vi "Installed Distributions [Hemanth].vi"() -> ()   [LabVIEW 2011]
uses:
  <vilib>/registry/registry.llb/Registry SAM.ctl
  <vilib>/registry/registry.llb/Read Registry Value Simple STR.vi
panel:
  in  "Searching in Registry Key and C:\\VM_SETUP\\scriptOut.log":string="SOFTWARE\\National Instruments\\Common\\Installer\\Distributions"
  out "Paths To Installers":string
  out "Dist Names":string[](array[string])
  out "Dist Paths":string[](array[string])
  out "error out":errorcluster
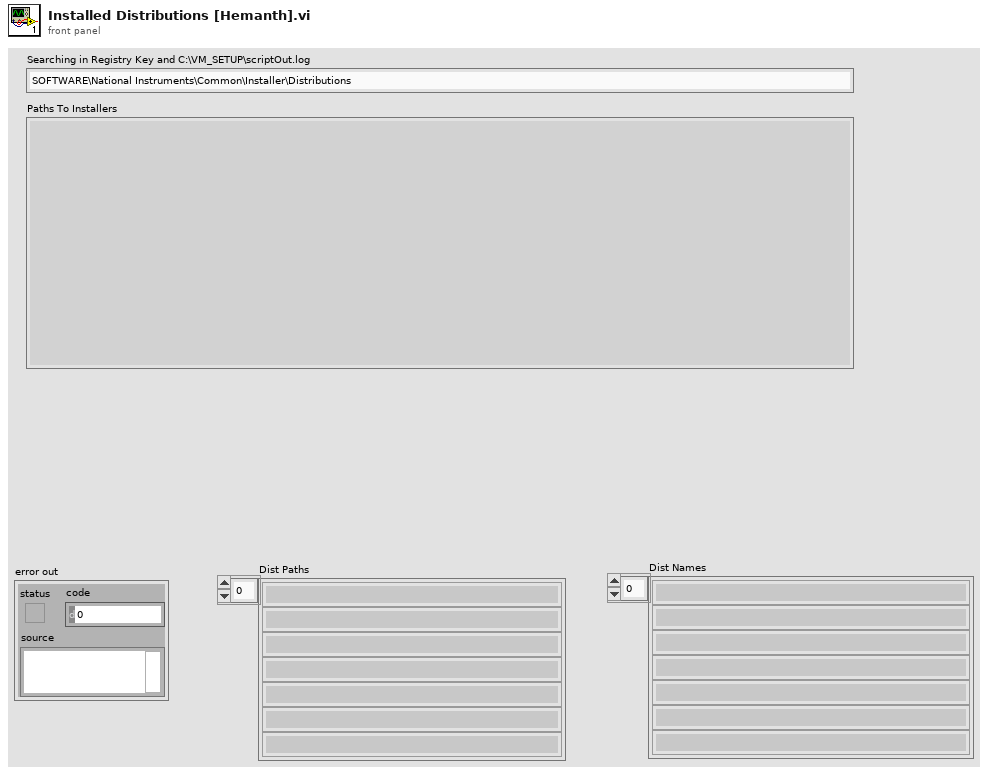
[diagram p1: front panel]
types:
  T1 = typedef "Registry SAM.ctl" = enum32{"KEY_QUERY_VALUE", "KEY_SET_VALUE", "KEY_CREATE_SUB_KEY", "KEY_ENUMERATE_SUB_KEYS", "KEY_NOTIFY", "KEY_CREATE_LINK", "KEY_READ", "KEY_WRITE", "KEY_ALL_ACCESS", "KEY_READ | KEY_WRITE"}
  T2 = typedef "Registry refnum.ctl" = refnum<k1>
  T3 = cluster{"numSubKeys":i32, "maxSubKeyLen":i32, "maxSubKeyClassLen":i32}
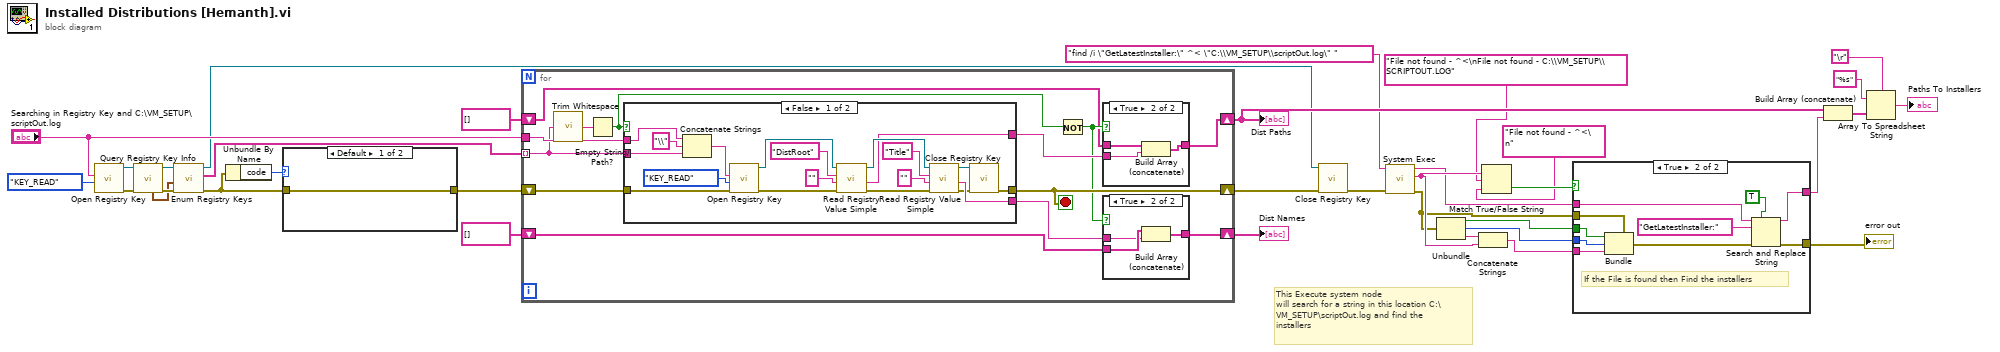
[diagram p0: block diagram]
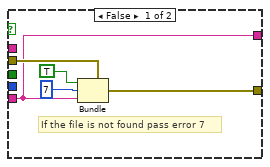
[diagram p2: hidden frame]
diagram:
  # "This Execute system node \nwill search for a string in this location C:\\VM_SETUP\\scriptOut.log and find the installers"
  n1 = call <vilib>:"Open Registry Key.vi"("security access mask (KEY_READ | KEY_WRITE)"=Registry_SAM."KEY_READ", "subkey"="Searching in Registry Key and C:\\VM_SETUP\\scriptOut.log") -> ("error out"=w27:errorcluster, "refnum out"=w29:T2)  [unwired: 8 in]
  n2 = call <vilib>:"Query Registry Key Info.vi"("error in (no error)"=w27, "refnum"=w29) -> ("error out"=w26:errorcluster, "refnum out"=w28:T2, "subkey info"=w25:T3)  [unwired: 5 in, 2 out]
  n3 = call <vilib>:"Enum Registry Keys.vi"("error in (no error)"=w26, "subkey info"=w25, "refnum"=w28) -> ("error out"=w30:errorcluster, "subkeys"=w34:string[], "refnum out"=w15:T2)  [unwired: 6 in]
  n4 = Unbundle By Name(w30) -> ("code"=w31:i32)
  n5 = case shown="Default" w31 {
    tunnel: [w36 _] -> w16
    tunnel: w30 -> [w36 _]
    frame Default {
    }
    frame -605 {
      # "This case is when you have \nless than 100 distirbutions\ninstalled"
    }
  }
  n6 = for {
    tunnel: w34 -> [w44] mode=indexing
    tunnel: "Searching in Registry Key and C:\\VM_SETUP\\scriptOut.log" -> [w49]
    shift-right: [w45] -> w14
    shift-left: w16 -> [w48]
    shift-right: [w39] -> w19
    shift-left: string[] [] ("Array") -> [w40]
    shift-right: [w37] -> w32
    shift-left: string[] [] ("Array") -> [w38]
    stop <- w45 stop-if-true
    n7 = call <vilib>:"Trim Whitespace.vi"("string"=w44) -> ("trimmed string"=w43:string)  [unwired: 1 in]
    n8 = Empty String/Path?(string/path=w43) -> (empty?=w42:bool)
    n9 = case shown="False" w42 {
      tunnel: w49 -> [w75 _]
      tunnel: w44 -> [w74 _]
      tunnel: w48 -> [w71 _]
      tunnel: [w63 _] -> w47
      tunnel: [w59 _] -> w45
      tunnel: [w61 _] -> w46
      frame False {
        n10 = Concatenate Strings(w75, "\\" ("string"), w74) -> (w73:string)
        n11 = call <vilib>:"Open Registry Key.vi"("error in (no error)"=w71, "security access mask (KEY_READ | KEY_WRITE)"=Registry_SAM."KEY_READ", "subkey"=w73) -> ("error out"=w70:errorcluster, "refnum out"=w67:T2)  [unwired: 7 in]
        n12 = call-poly <vilib>:"Read Registry Value Simple.vi"("error in (no error)"=w70, "default data"="", "value"="DistRoot", "refnum"=w67) -> ("error out"=w62:errorcluster, "String/Binary data"=w63:string, "refnum out"=w66:T2)  [unwired: 2 in, 1 out]
        n13 = call-poly <vilib>:"Read Registry Value Simple.vi"("error in (no error)"=w62, "default data"="", "value"="Title", "refnum"=w66) -> ("error out"=w60:errorcluster, "String/Binary data"=w61:string, "refnum out"=w58:T2)  [unwired: 2 in, 1 out]
        n14 = call <vilib>:"Close Registry Key.vi"("error in (no error)"=w60, "refnum"=w58) -> ("error out"=w59:errorcluster)  [unwired: 5 in]
      }
      frame True {
      }
    }
    n15 = Not(x=w42) -> (.not. x?=w41:bool)
    n16 = case shown="True" w41 {
      tunnel: w40 -> [w54 w56]
      tunnel: w47 -> [_ w55]
      tunnel: [w54 w57] -> w39
      frame False {
      }
      frame True {
        n17 = Build Array (concatenate)(w56, w55) -> (w57:string[])
      }
    }
    n18 = case shown="True" w41 {
      tunnel: w38 -> [w50 w52]
      tunnel: w46 -> [_ w51]
      tunnel: [w50 w53] -> w37
      frame False {
      }
      frame True {
        n19 = Build Array (concatenate)(w52, w51) -> (w53:string[])
      }
    }
  }
  "Dist Paths" <- w19
  "Dist Names" <- w32
  n20 = call <vilib>:"Close Registry Key.vi"("error in (no error)"=w14, "refnum"=w15) -> ("error out"=w13:errorcluster)  [unwired: 5 in]
  n21 = call <vilib>:"System Exec.vi"("error in (no error)"=w13, "command line"="find /i \"GetLatestInstaller:\" ^< \"C:\\VM_SETUP\\scriptOut.log\" ") -> ("error out"=w6:errorcluster, "standard error"=w11:string, "standard output"=w10:string)  [unwired: 6 in, 1 out]
  n22 = Unbundle(w6) -> ("status"=w5:bool, "code"=w4:i32, "source"=w12:string)
  n23 = Concatenate Strings(w12, w11) -> (w3:string)
  n24 = Match True/False String(2:"File not found - ^<\n" ("false string"), 3:"File not found - ^<\nFile not found - C:\\VM_SETUP\\SCRIPTOUT.LOG" ("true string"), 4:w11) -> (0:w9:bool)  [unwired: 1 out]
  n25 = case shown="True" w9 {
    tunnel: w10 -> [_ w91]
    tunnel: [w77 w82] -> w1
    tunnel: w6 -> [w81 w88]
    tunnel: w5 -> [_ w87]
    tunnel: w4 -> [_ w86]
    tunnel: w3 -> [w77 w85]
    tunnel: [w80 w83] -> w2
    frame False {
      # "If the file is not found pass error 7"
      n26 = Bundle(cluster=w81, "status"=TRUE, "code"=7, "source"=w77) -> (w80:errorcluster)
    }
    frame True {
      # "If the File is found then Find the installers"
      n27 = Bundle(cluster=w88, "status"=w87, "code"=w86, "source"=w85) -> (w84:errorcluster)
      n28 = Search and Replace String(replace all?=TRUE ("replace all? (F)"), input string=w91, search string="GetLatestInstaller:", error in=w84) -> (result string=w82:string, error out=w83:errorcluster)  [unwired: 4 in, 2 out]
    }
  }
  "error out" <- w2
  n29 = Build Array (concatenate)(w19, w1) -> (w18:string[])
  n30 = Array To Spreadsheet String(delimiter (Tab)="\r", array=w18, 3:"%s" ("format string")) -> (spreadsheet string=→"Paths To Installers":string)
